vi "Queue Is Nested.vi"(10 "Alias":string, 11 "Base Event jettl in":refnum<class "Base Event jettl.lvclass">) -> (2 "Queue Is Nested?":bool)   [LabVIEW 2021, in "jettl.lvlib" / "Base Event jettl.lvlib" / "Base Event jettl.lvclass"]
uses:
  Base Event jettl.lvclass
  Base Event jettl.lvclass/Base Event jettl.ctl
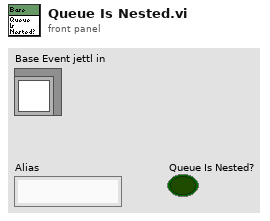
[diagram p1: front panel]
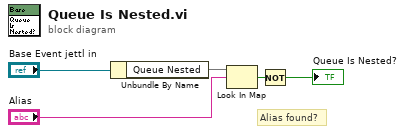
[diagram p0: block diagram]
diagram:
  # "Alias found?"
  n1 = Unbundle By Name("Base Event jettl in") -> ("Queue Nested"=w5:map{string, refnum<data-value>})
  n2 = Look In Map(map=w5, key="Alias") -> (key not found?=w4:bool)  [unwired: 1 in, 1 out]
  n3 = Not(x=w4) -> (.not. x?=→"Queue Is Nested?":bool)
